vi "4.5.vi"() -> ()   [LabVIEW 2017]
panel:
  out "随机数":i32
  in  "指定值":dbl
  out "循环次数":i32
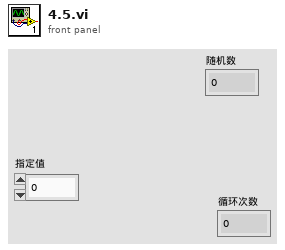
[diagram p1: front panel]
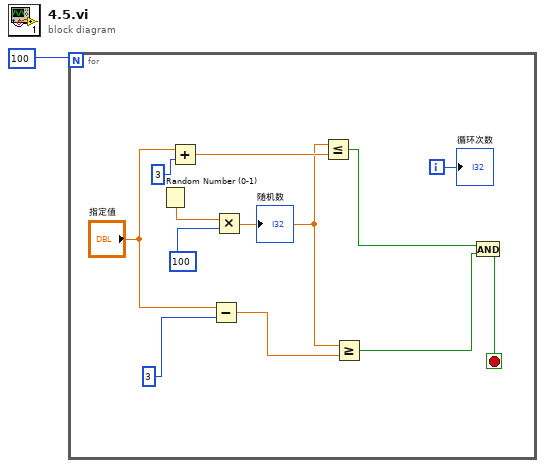
[diagram p0: block diagram]
diagram:
  n1 = for {
    N: 100 -> [_]
    i -> [w13]
    stop <- w3 stop-if-true
    n2 = Random Number (0-1)() -> (number: 0 to 1=w12:dbl)
    n3 = Add(x="指定值", y=3) -> (x+y=w7:dbl)
    n4 = Subtract(x="指定值", y=3) -> (x-y=w6:dbl)
    n5 = Multiply(x=w12, y=100) -> (x*y=w2:dbl)
    "随机数" <- w2
    n6 = Less Or Equal?(x=w2, y=w7) -> (x <= y?=w5:bool)
    n7 = Greater Or Equal?(x=w2, y=w6) -> (x >= y?=w4:bool)
    n8 = And(x=w5, y=w4) -> (x .and. y?=w3:bool)
    "循环次数" <- w13
  }
